vi "local.Connect.vi"(0 "SLSC Local in":refnum<class "SLSC Interface.lvclass">, 5 "devices":refnum<k21>="$DefaultDevices", 11 "error in (no error)":errorcluster, 12 "connect timeout (60 sec)":dbl=60.0) -> (4 "SLSC Local out":refnum<class "SLSC Interface.lvclass">, 15 "error out":errorcluster)   [LabVIEW 2016, in "SLSC Interfaces.lvlib" / "SLSC Interface.lvclass"]
uses:
  SLSC Interface Class/SLSC Interface.lvclass
  <vilib>/SLSC/SLSC.lvlib
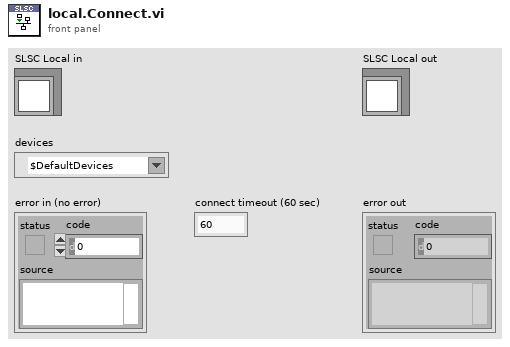
[diagram p1: front panel]
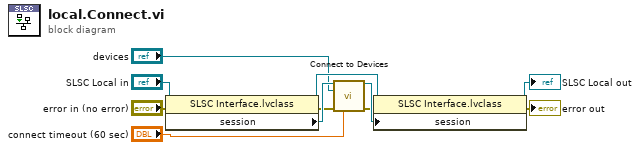
[diagram p0: block diagram]
diagram:
  n1 = property class="SLSC Interface.lvclass"(reference="SLSC Local in", error in="error in (no error)") -> (reference out=w11:refnum<class "SLSC Interface.lvclass">, error out=w9:errorcluster, "session"=w10:refnum<k21>)
  n2 = call <vilib>:"Connect to Devices.vi"("session in"=w10, "devices"="devices", "error in (no error)"=w9, "connect timeout (60 sec)"="connect timeout (60 sec)") -> ("session out"=w8:refnum<k21>, "error out"=w7:errorcluster)  [unwired: 10 in]
  n3 = property class="SLSC Interface.lvclass"(reference=w11, error in=w7, "session"=w8) -> (reference out=→"SLSC Local out":refnum<class "SLSC Interface.lvclass">, error out=→"error out":errorcluster)
